vi "Phasor Compute tau_phi & tau_m from Phasor (Discrete, Gated).vi"(8 "Error In":errorcluster, 9 "Phasor L_N[W] Parameters":T1, 10 "max tau":dbl[unit], 11 "Phasor":cluster{"X":dbl, "Y":dbl}) -> (0 "Error Out":errorcluster, 1 "Modulus Lifetime":dbl[unit], 3 "Phase Lifetime":dbl[unit], 5 "Modulus Lifetime Zeros":dbl[](array[numeric]) format="%.2f", 7 "Phase Lifetime Zeros":dbl[](array[numeric]) format="%.2f")   [LabVIEW 2021, in "Phasor.lvlib"]
uses:
  Phasor.lvlib
  Phasor L_N[W] Parameters.ctl
  Phasor tau_phi & tau_m Zero Finder Parameters.ctl
  Phasor Explorer Zero Finder tau (Discrete, Gated Phasor).vi
  <vilib>/gmath/zero.llb/Find All Zeros of f(x) (VI).vi
  <vilib>/gmath/NI_Gmath.lvlib
  Phasor Explorer.lvlib
  Error/Error.lvlib
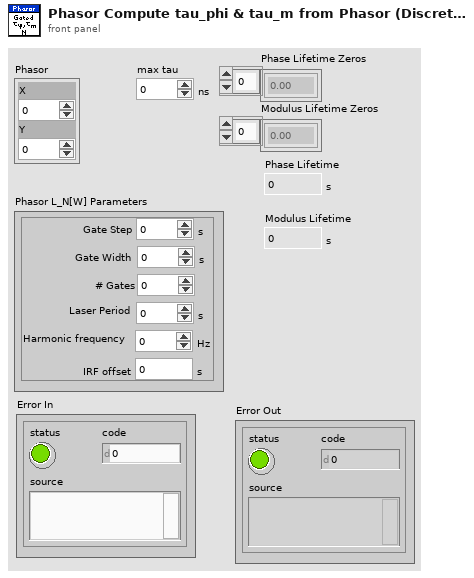
[diagram p1: front panel]
types:
  T1 = typedef "Phasor.lvlib/Phasor L_N[W] Parameters.ctl" = cluster{"Laser Period":dbl[unit], "Gate Width":dbl[unit], "Gate Step":dbl[unit], "Harmonic frequency":dbl[unit], "IRF offset":dbl[unit], "# Gates":dbl}
  T2 = typedef "Phasor.lvlib/Phasor tau_phi & tau_m Zero Finder Parameters.ctl" = cluster{"Period":ext, "Width":ext, "# Gates":ext, "f":ext, "tan(phi), m":ext, "phi(T)/m(F)":bool, "Offset":ext}
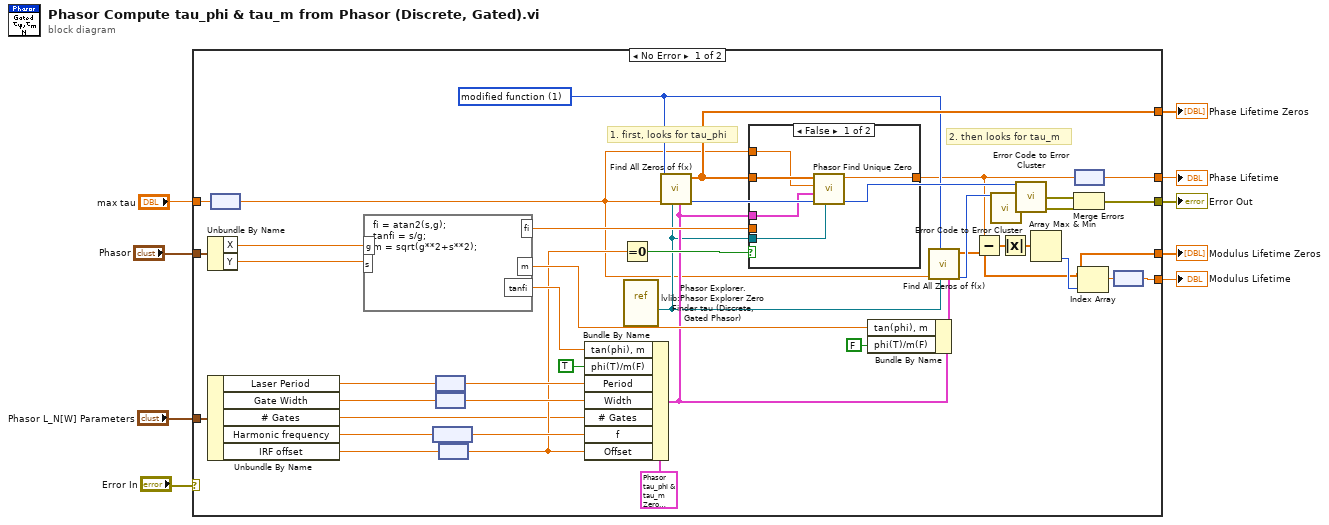
[diagram p0: block diagram]
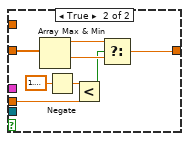
[diagram p2: hidden frame]
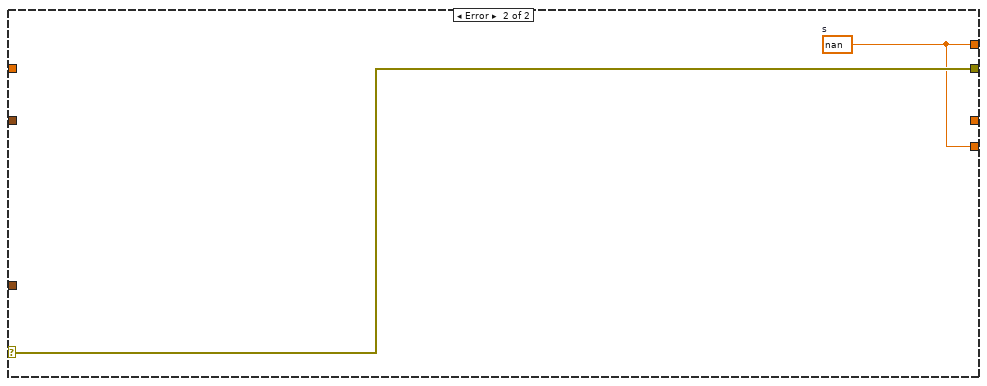
[diagram p3: hidden frame]
diagram:
  n1 = case shown="No Error" "Error In" {
    selector: "Error In" -> [_ w64]
    tunnel: "max tau" -> [w49 _]
    tunnel: [w48 _] -> w8
    tunnel: "Phasor" -> [w47 _]
    tunnel: [w38 w63] -> w6
    tunnel: [w34 w64] -> w5
    tunnel: [w32 w63] -> w4
    tunnel: [w27 _] -> w3
    tunnel: "Phasor L_N[W] Parameters" -> [w17 _]
    frame No Error {
      w33 = u16 1 items=["fixed function", "modified function"] ("step type")
      # "2. then looks for tau_m"
      # "1. first, looks for tau_phi"
      n2 = Unbundle By Name(w47) -> ("X"=w46:dbl, "Y"=w45:dbl)
      n3 = Unbundle By Name(w17) -> ("Laser Period"=w16:dbl[unit], "Gate Width"=w15:dbl[unit], "# Gates"=w12:dbl, "Harmonic frequency"=w14:dbl[unit], "IRF offset"=w13:dbl[unit])
      n4 = node(w49) -> (w18:dbl)
      n5 = formula code="fi = atan2(s,g);\ntanfi = s/g;\nm = sqrt(g**2+s**2);"("g"=w46, "s"=w45) -> ("tanfi"=w25:dbl, "m"=w39:dbl, "fi"=w22:dbl)
      n6 = node(w14) -> (w42:dbl)
      n7 = node(w16) -> (w44:dbl)
      n8 = node(w15) -> (w43:dbl)
      n9 = node(w13) -> (w23:dbl)
      n10 = Bundle By Name(cluster=T2 {"Period"=0.0, "Width"=0.0, "# Gates"=0.0, "f"=0.0, "tan(phi), m"=0.0, "phi(T)/m(F)"=TRUE, "Offset"=0.0}, "tan(phi), m"=w25, "phi(T)/m(F)"=TRUE, "Period"=w44, "Width"=w43, "# Gates"=w12, "f"=w42, "Offset"=w23) -> (w20:T2)
      n11 = Equal To 0?(x=w23) -> (x = 0?=w21:bool)
      n12 = vi-ref "Phasor Explorer.lvlib:Phasor Explorer Zero Finder tau (Discrete, Gated Phasor).vi"() -> (w19:refnum<vi>)
      n13 = call-poly <vilib>:"Find All Zeros of f(x).vi"("data"=w20, "f(x)"=w19, "end"=w18, "step type"=w33) -> ("error"=w36:i32, "Zeros"=w48:dbl[])  [unwired: 4 in, 2 out]
      n14 = case shown="False" w21 {
        tunnel: w48 -> [w53 w62]
        tunnel: [w54 w59] -> w31
        tunnel: w22 -> [_ w58]
        tunnel: w20 -> [w51 _]
        tunnel: w19 -> [w50 _]
        tunnel: w18 -> [w52 _]
        frame False {
          n15 = call "Phasor Find Unique Zero.vi"("VI in"=w50, "Zero Finder Parameters"=w51, "max tau"=w52, "Zeros"=w53) -> ("Phase Lifetime"=w54:dbl)  [unwired: 6 in, 1 out]
        }
        frame True {
          n16 = Array Max & Min(array=w62) -> (max value=w61:dbl, min value=w60:dbl)  [unwired: 2 out]
          n17 = Negate(x=1.5707963267948966) -> (-x=w55:dbl)
          n18 = Less?(x=w55, y=w58) -> (x < y?=w57:bool)
          n19 = Select(t=w61, s=w57, f=w60) -> (s? t:f=w59:dbl)
        }
      }
      n20 = Bundle By Name(cluster=w20, "tan(phi), m"=w39, "phi(T)/m(F)"=FALSE) -> (w37:T2)
      n21 = call-poly <vilib>:"Find All Zeros of f(x).vi"("data"=w37, "f(x)"=w19, "end"=w18, "step type"=w33) -> ("error"=w35:i32, "Zeros"=w27:dbl[])  [unwired: 4 in, 2 out]
      n22 = Subtract(x=w31, y=w27) -> (x-y=w30:dbl[])
      n23 = call "Error Code to Error Cluster.vi"("Error Code"=w35) -> ("Error Out"=w10:errorcluster)  [unwired: 14 in]
      n24 = Absolute Value(x=w30) -> (abs(x)=w29:dbl[])
      n25 = call "Error Code to Error Cluster.vi"("Error Code"=w36) -> ("Error Out"=w11:errorcluster)  [unwired: 14 in]
      n26 = Array Max & Min(array=w29) -> (min index (indices)=w28:i32)  [unwired: 3 out]
      n27 = Merge Errors(w11, w10) -> (w34:errorcluster)
      n28 = node(w31) -> (w32:dbl[unit])
      n29 = Index Array(array=w27, index=w28) -> (element=w26:dbl)
      n30 = node(w26) -> (w38:dbl[unit])
    }
    frame Error {
      w63 = dbl[unit] nan  # s
    }
  }
  "Modulus Lifetime" <- w6
  "Phase Lifetime" <- w4
  "Error Out" <- w5
  "Phase Lifetime Zeros" <- w8
  "Modulus Lifetime Zeros" <- w3
